vi "FindItem.vi"(7 "Item Name":string, 8 "error in (no error)":errorcluster, 10 "StructuredDataContainer":variant, 11 "BlueSerializer in":refnum<class "BlueSerializer.lvclass">) -> (0 "error out":errorcluster, 1 "Found?":bool, 2 "StructuredDataItem":variant, 3 "BlueSerializer out":refnum<class "BlueSerializer.lvclass">)   [LabVIEW 2019, in "BlueSerialization.lvlib" / "BlueSerializer.lvclass"]
uses:
  BlueSerializer.lvclass
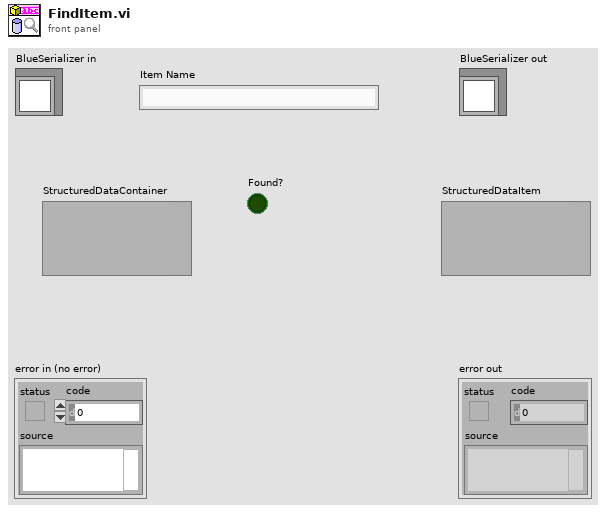
[diagram p1: front panel]
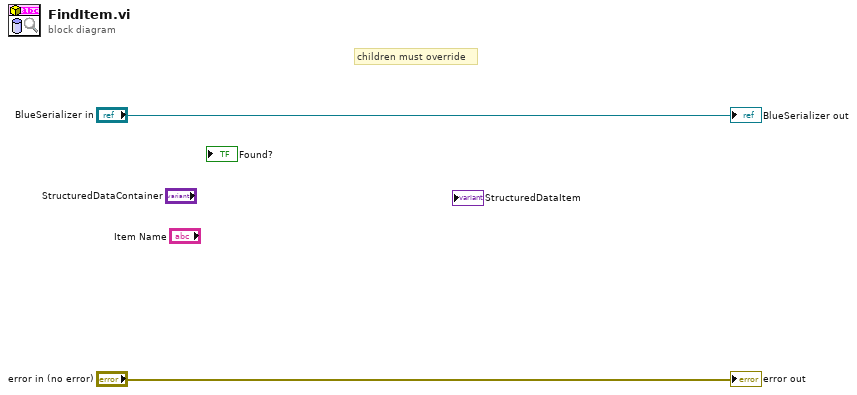
[diagram p0: block diagram]
diagram:
  # "children must override"
  "error out" <- "error in (no error)"
  "BlueSerializer out" <- "BlueSerializer in"
